vi "ep_Scaling Sensitivity.vi"(8 "error in (no error)":errorcluster, 9 "system info in":refnum<class "EP System Info.lvclass">, 10 "sensitivity":dbl[](array[numeric]), 11 "waveforms in":waveform(dbl)[](array[waveform])) -> (0 "error out":errorcluster, 1 "system info out":refnum<class "EP System Info.lvclass">, 3 "waveforms out":waveform(dbl)[](array[waveform]))   [LabVIEW 2014, in "NI_EP_Power Quality.lvlib"]
uses:
  <vilib>/addons/Electrical Power/PQ/NI_EP_Power Quality.lvlib
  <vilib>/addons/Electrical Power/PQ/Common/Classes/System Info/EP System Info.lvclass
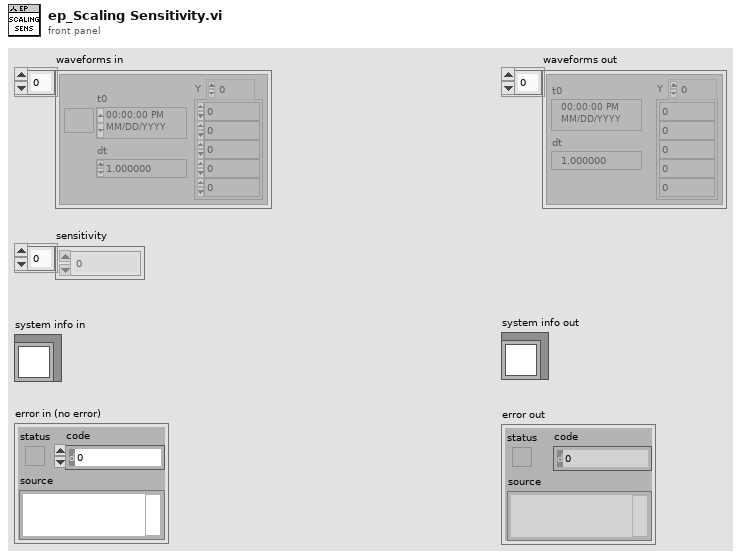
[diagram p1: front panel]
types:
  T1 = typedef "NI_EP_Power Quality.lvlib/ep_Channel Sensitivity.ctl" = cluster{"3-phase system ID":string, "sensitivity":dbl[]}
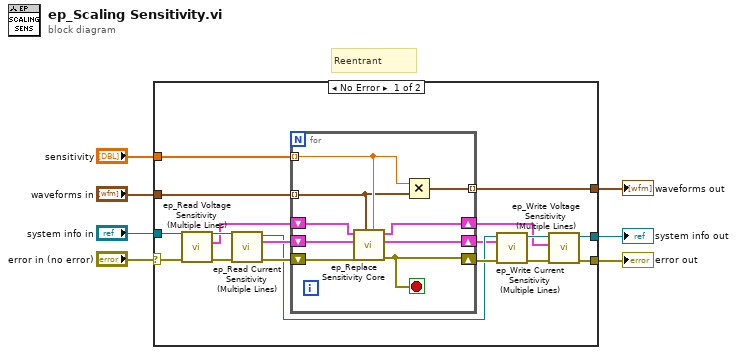
[diagram p0: block diagram]
diagram:
  # "Reentrant"
  n1 = case shown="No Error" "error in (no error)" {
    selector: "error in (no error)" -> [w20 w36]
    tunnel: "system info in" -> [w24 w35]
    tunnel: [w14 w35] -> w6
    tunnel: [w11 w36] -> w5
    tunnel: [w19 _] -> w1
    tunnel: "waveforms in" -> [w18 _]
    tunnel: "sensitivity" -> [w17 _]
    frame No Error {
      n2 = call <vilib>:"ep_Read Voltage Sensitivity (Multiple Lines).vi"("error in (no error)"=w20, "system info in"=w24) -> ("error out"=w22:errorcluster, "voltage sensitivity (multiline)"=w16:T1[], "system info out"=w25:refnum<class "EP System Info.lvclass">)  [unwired: 7 in]
      n3 = call <vilib>:"ep_Read Current Sensitivity (Multiple Lines).vi"("error in (no error)"=w22, "system info in"=w25) -> ("error out"=w21:errorcluster, "current sensitivity (multiline)"=w23:T1[], "system info out"=w10:refnum<class "EP System Info.lvclass">)  [unwired: 7 in]
      n4 = for {
        shift-right: [w29] -> w13
        shift-left: w21 -> [w32]
        tunnel: [w34] -> w19 mode=indexing
        tunnel: w18 -> [w30] mode=indexing
        tunnel: w17 -> [w31] mode=indexing
        shift-right: [w26] -> w9
        shift-left: w23 -> [w33]
        shift-right: [w27] -> w8
        shift-left: w16 -> [w28]
        stop <- w29 stop-if-true
        n5 = call <vilib>:"ep_Replace Sensitivity Core.vi"("sensitivity"=w31, "waveform"=w30, "error in (no error)"=w32, "current sensitivity (multiline) in"=w33, "voltage sensitivity (multiline) in"=w28) -> ("error out"=w29:errorcluster, "current sensitivity (multiline) out"=w26:T1[], "voltage sensitivity (multiline) out"=w27:T1[])  [unwired: 4 in]
        n6 = Multiply(x=w31, y=w30) -> (x*y=w34:waveform(dbl))
      }
      n7 = call <vilib>:"ep_Write Current Sensitivity (Multiple Lines).vi"("error in (no error)"=w13, "current sensitivity (multiline)"=w9, "system info in"=w10) -> ("error out"=w12:errorcluster, "system info out"=w15:refnum<class "EP System Info.lvclass">)  [unwired: 7 in]
      n8 = call <vilib>:"ep_Write Voltage Sensitivity (Multiple Lines).vi"("error in (no error)"=w12, "voltage sensitivity (multiline)"=w8, "system info in"=w15) -> ("error out"=w11:errorcluster, "system info out"=w14:refnum<class "EP System Info.lvclass">)  [unwired: 7 in]
    }
    frame Error {
    }
  }
  "error out" <- w5
  "system info out" <- w6
  "waveforms out" <- w1
